vi "logError.vi"(8 "Clear error?":bool=TRUE, 9 "Error to log":errorcluster, 10 "Location":string="Unknown", 11 "Text reference":refnum<vi>) -> (1 "error out":errorcluster)   [LabVIEW 2017]
uses:
  <vilib>/Utility/error.llb/DialogType.ctl
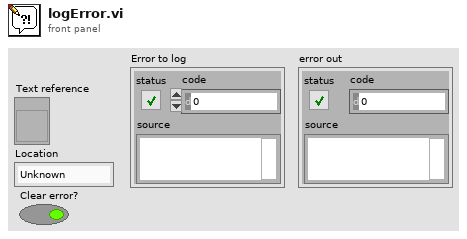
[diagram p1: front panel]
types:
  T1 = typedef "DialogType.ctl" = u16
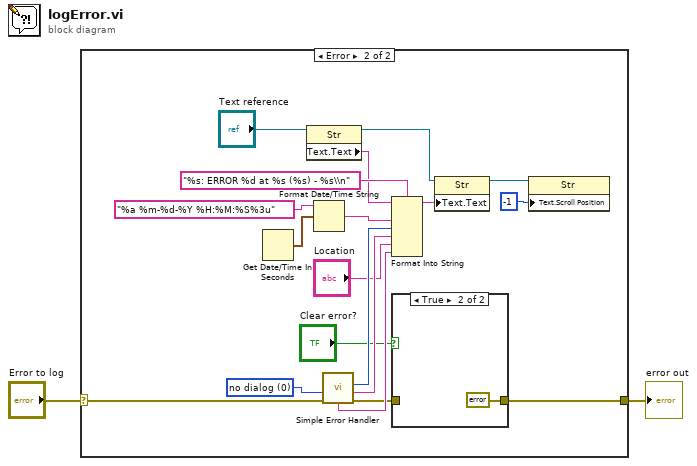
[diagram p0: block diagram]
diagram:
  n1 = case shown="Error" "Error to log" {
    selector: "Error to log" -> [w3 w11]
    tunnel: [w3 w4] -> w1
    frame No Error {
    }
    frame Error {
      w12 = T1 0 items=["no dialog", "OK message", "continue or stop message", "OK message + warnings", "continue/stop + warnings"] ("type of dialog (OK msg:1)")
      n2 = Get Date/Time In Seconds() -> (seconds since 1Jan1904=w22:timestamp)
      n3 = property class="Str"(reference="Text reference") -> (reference out=w14:refnum<vi>, "Text.Text"=w16:string)  [unwired: 1 in, 1 out]
      n4 = Format Date/Time String(time format string (%c)="%a %m-%d-%Y %H:%M:%S%3u", seconds (now)=w22) -> (date/time string=w20:string)  [unwired: 1 in]
      n5 = call <vilib>:"Simple Error Handler.vi"("type of dialog (OK msg:1)"=w12, "error in (no error)"=w11) -> ("code out"=w10:i32, "source out"=w9:string, "error out"=w5:errorcluster, "message"=w8:string)  [unwired: 3 in, 1 out]
      n6 = Format Into String(format string="%s: ERROR %d at %s (%s) - %s\\n", initial string=w16, w20, w10, w9, "Location", w8) -> (resulting string=w17:string)  [unwired: 1 in, 1 out]
      n7 = case shown="True" "Clear error?" {
        tunnel: [w23 errorcluster {"status"=FALSE, "code"=0, "source"=""} ("error out")] -> w4
        tunnel: w5 -> [w23 _]
        frame False {
        }
        frame True {
        }
      }
      n8 = property class="Str"(reference=w14, "Text.Text"=w17) -> (reference out=w15:refnum<vi>)  [unwired: 1 in, 1 out]
      n9 = property class="Str"(reference=w15, "Text.Scroll Position"=-1) -> ()  [unwired: 1 in, 2 out]
    }
  }
  "error out" <- w1
